vi "Parse TOML String.vi"(8 "error in (no error)":errorcluster, 11 "String":string) -> (0 "error out":errorcluster, 3 "Value":T1)   [LabVIEW 2019, in "BlueTOMLSerializer.lvlib"]
uses:
  BlueTOMLSerializer.lvlib
  Context.ctl
  State.ctl
  <vilib>/regexp/Match Regular Expression.xnode
  Value.ctl
  Key-Value Pair.ctl
  Table Context.ctl
  Array Context.ctl
  Table Array Context.ctl
  TOML Value.ctl
  Value Type.ctl
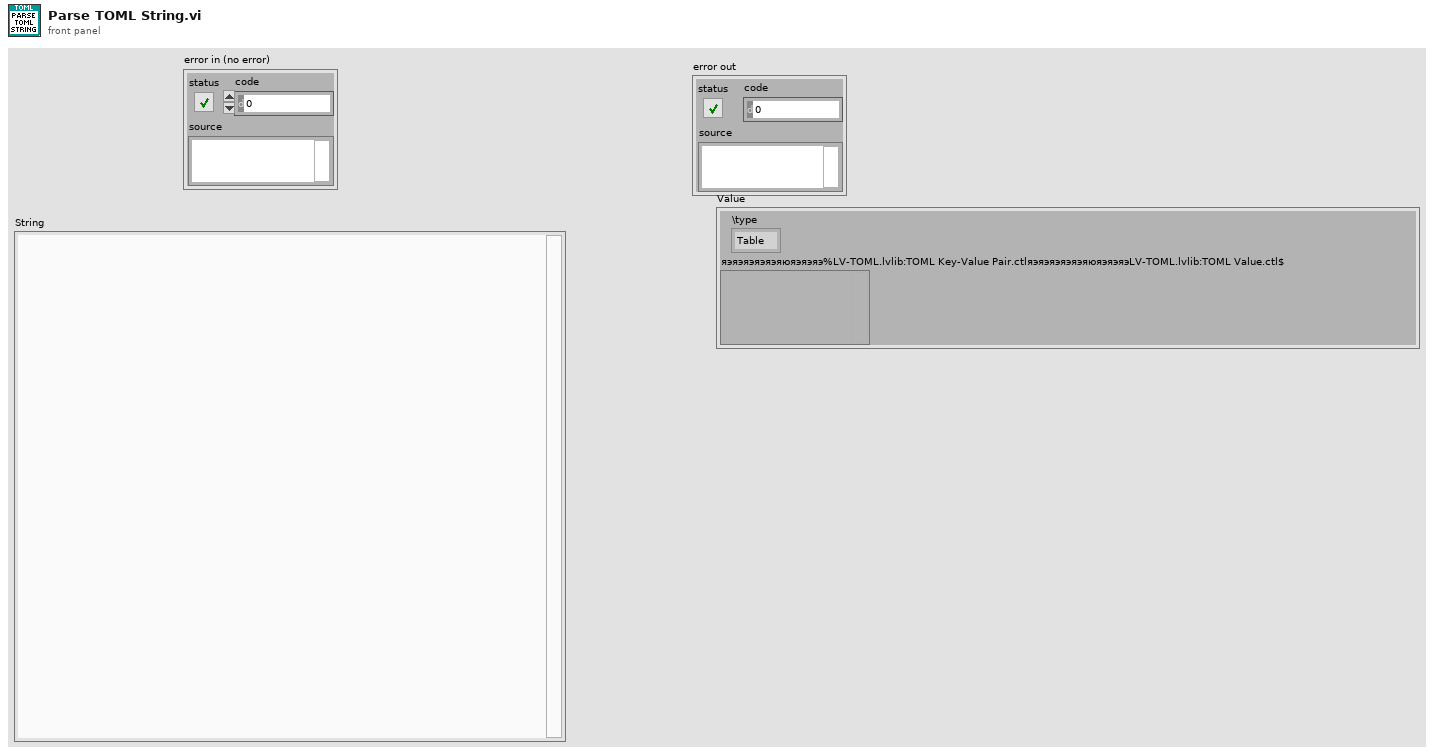
[diagram p1: front panel]
types:
  T1 = typedef "BlueTOMLSerializer.lvlib/TOML Value.ctl" = cluster{"\\type":enum16{"Table", "Array", "String", "Integer", "Float", "Boolean", "Offset Date-Time", "Local Date-Time", "Local Date", "Local Time"}, "яэяэяэяэяэяюяэяэяэ%LV-TOML.lvlib:TOML Key-Value Pair.ctlяэяэяэяэяэяюяэяэяэLV-TOML.lvlib:TOML Value.ctl$":variant}
  T2 = typedef "BlueTOMLSerializer.lvlib/Key-Value Pair.ctl" = cluster{"Key":string, "Value":T3}
  T3 = typedef "BlueTOMLSerializer.lvlib/Value.ctl" = cluster{"Type":T4, "Value":variant}
  T4 = typedef "BlueTOMLSerializer.lvlib/Value Type.ctl" = enum16{"Table", "Array", "String", "Integer", "Float", "Boolean", "Offset Date-Time", "Local Date-Time", "Local Date", "Local Time"}
  T5 = enum16{"Table", "Array", "String", "Integer", "Float", "Boolean", "Offset Date-Time", "Local Date-Time", "Local Date", "Local Time"}
  T6 = typedef "BlueTOMLSerializer.lvlib/Table Context.ctl" = cluster{"Table":T2[], "Key":string, "Defined Keys":string[]}
  T7 = typedef "BlueTOMLSerializer.lvlib/Context.ctl" = cluster{"Type":enum16{"Table", "Array", "Inline Table", "Table Array"}, "Value":variant}
  T8 = typedef "BlueTOMLSerializer.lvlib/State.ctl" = enum16{"Table", "Value", "Inline Table"}
  T9 = typedef "BlueTOMLSerializer.lvlib/Table Array Context.ctl" = cluster{"Table Array":cluster{"Table":T2[]}[], "Index":i32, "Key":string}
  T10 = typedef "BlueTOMLSerializer.lvlib/Array Context.ctl" = cluster{"Array":T3[], "Index":i32, "Empty":bool, "Type":T4}
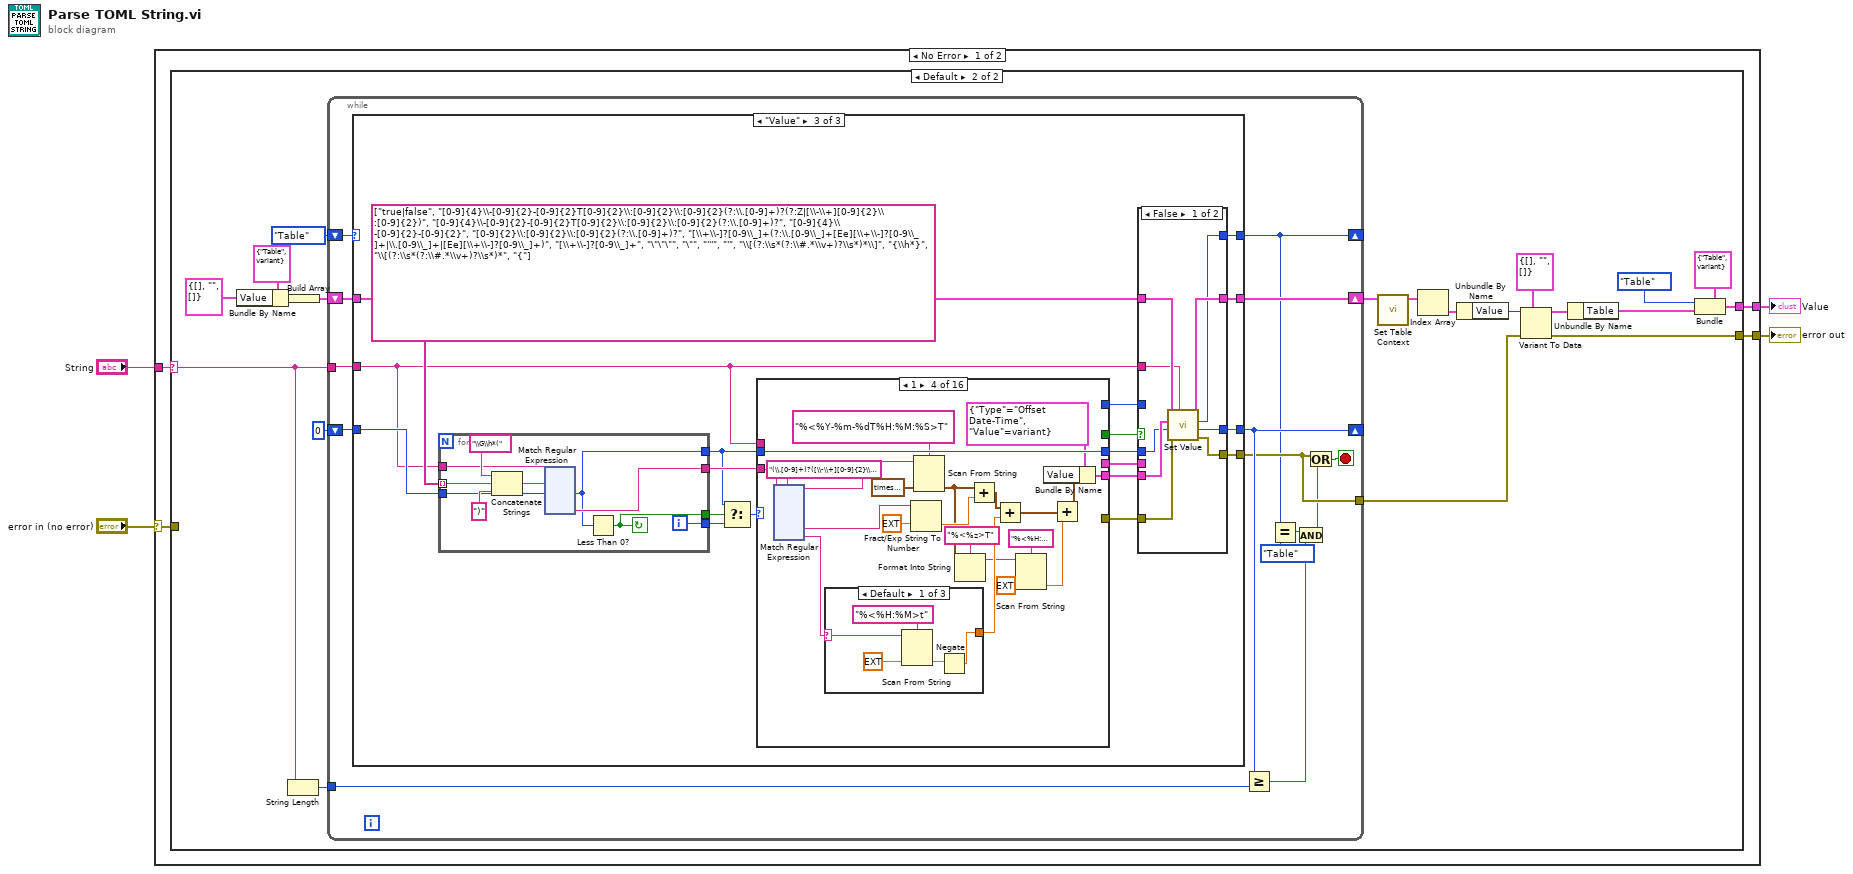
[diagram p0: block diagram]
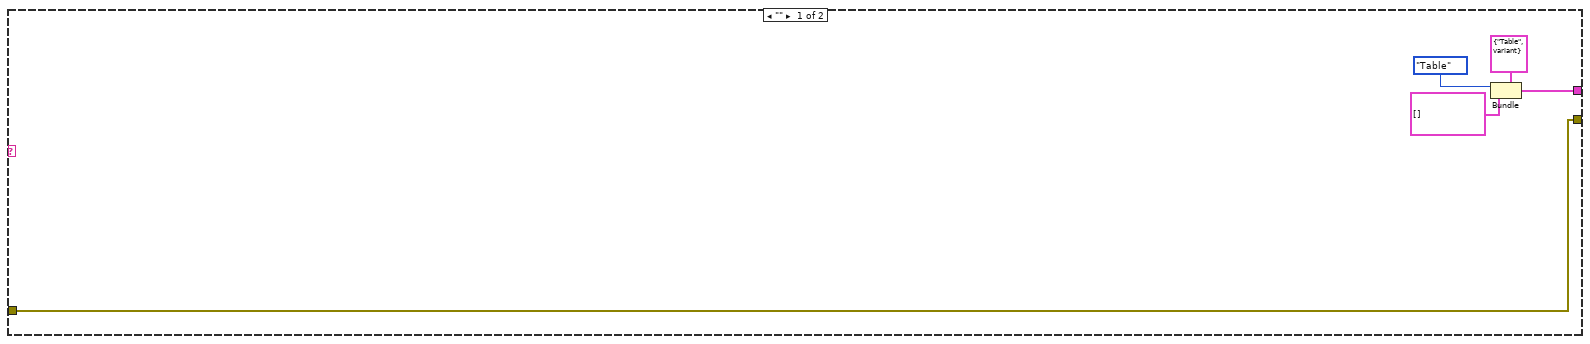
[diagram p2: hidden frame]
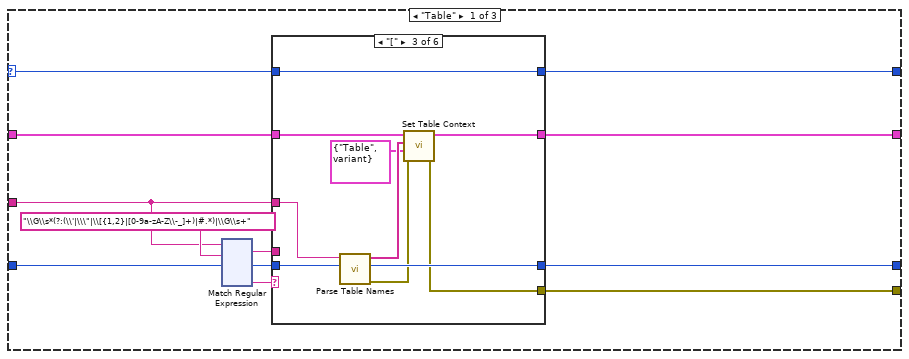
[diagram p3: hidden frame]
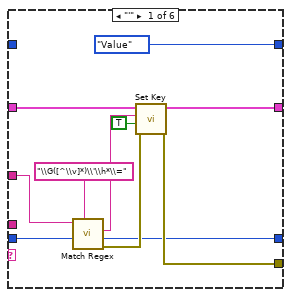
[diagram p4: hidden frame]
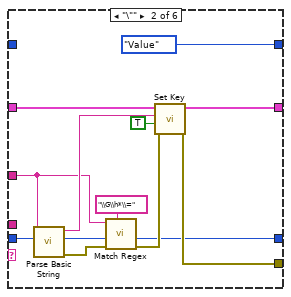
[diagram p5: hidden frame]
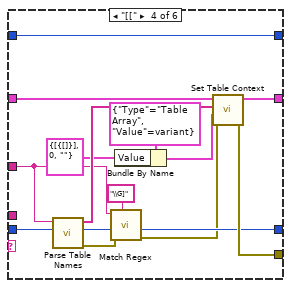
[diagram p6: hidden frame]
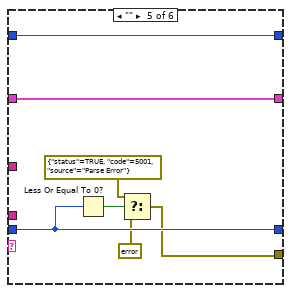
[diagram p7: hidden frame]
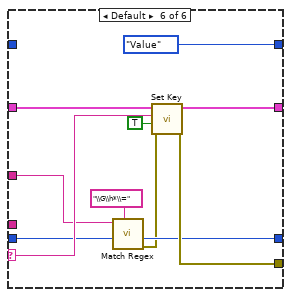
[diagram p8: hidden frame]
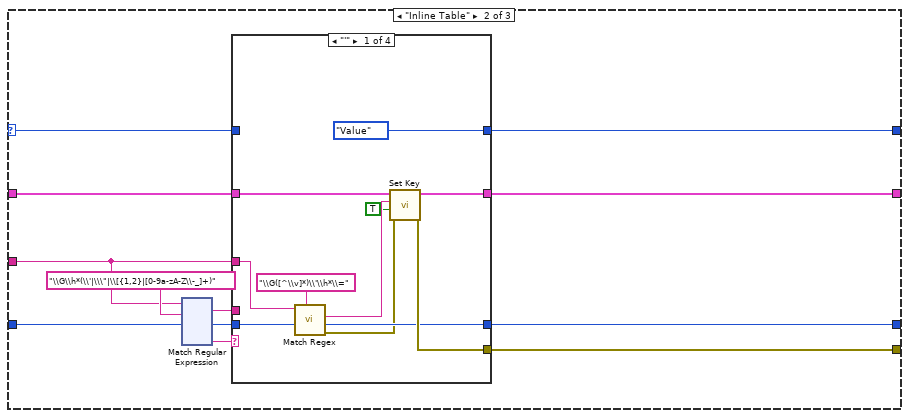
[diagram p9: hidden frame]
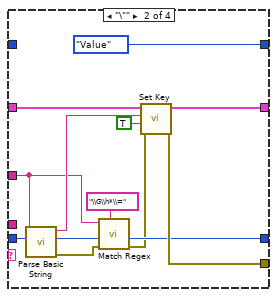
[diagram p10: hidden frame]
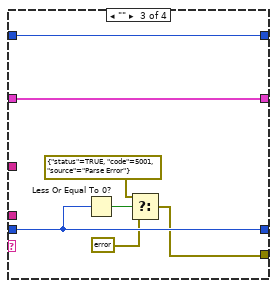
[diagram p11: hidden frame]
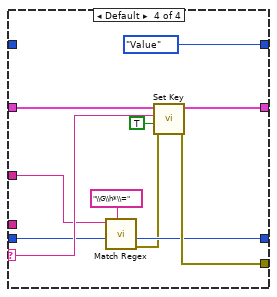
[diagram p12: hidden frame]
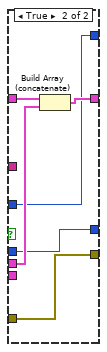
[diagram p13: hidden frame]
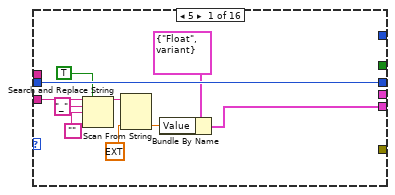
[diagram p14: hidden frame]
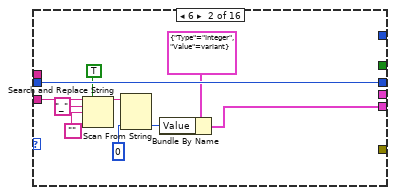
[diagram p15: hidden frame]
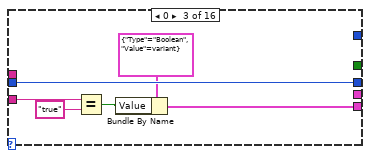
[diagram p16: hidden frame]
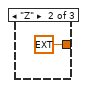
[diagram p17: hidden frame]
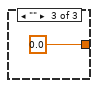
[diagram p18: hidden frame]
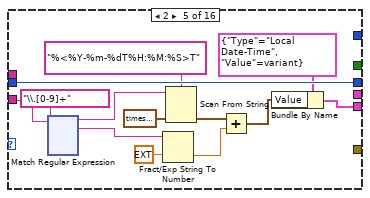
[diagram p19: hidden frame]
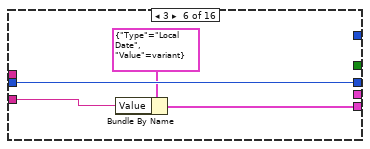
[diagram p20: hidden frame]
diagram:
  n1 = case shown="No Error" "error in (no error)" {
    selector: "error in (no error)" -> [w5 w930]
    tunnel: "String" -> [w8 _]
    tunnel: [w6 _] -> w1
    tunnel: [w7 w930] -> w3
    frame No Error {
      n2 = case shown="Default" w8 {
        selector: w8 -> [_ w31]
        tunnel: [w13 w23] -> w7
        tunnel: [w9 w18] -> w6
        tunnel: w5 -> [w13 _]
        frame "" {
          n3 = Bundle(cluster=T1 {"\\type"=enum."Table", "яэяэяэяэяэяюяэяэяэ%LV-TOML.lvlib:TOML Key-Value Pair.ctlяэяэяэяэяэяюяэяэяэLV-TOML.lvlib:TOML Value.ctl$"=variant} ("Value"), "\\type"=T5."Table" ("Type"), "яэяэяэяэяэяюяэяэяэ%LV-TOML.lvlib:TOML Key-Value Pair.ctlяэяэяэяэяэяюяэяэяэLV-TOML.lvlib:TOML Value.ctl$"=T2[] [] ("Table")) -> (w9:T1)
        }
        frame Default {
          n4 = Bundle By Name(cluster=T7 {"Type"=enum."Table", "Value"=variant} ("Context"), "Value"=T6 {"Table"=[], "Key"="", "Defined Keys"=[]} ("Table Context")) -> (w15:T7)
          n5 = String Length(string=w31) -> (length=w30:i32)
          n6 = Build Array(w15) -> (w14:T7[])
          n7 = while {
            tunnel: w31 -> [w46]
            shift-right: [w36] -> _
            shift-left: State."Table" ("State") -> [w47]
            shift-right: [w44] -> w29
            shift-left: w14 -> [w43]
            shift-right: [w39] -> _
            shift-left: 0 -> [w45]
            tunnel: w30 -> [w41]
            tunnel: [w38] -> w22
            stop <- w42 stop-if-true
            n8 = case shown="\"Value\"" w47 {
              selector: w47 -> [w55 w250 _]
              tunnel: w46 -> [w49 w244 w413]
              tunnel: w45 -> [w48 w243 w430]
              tunnel: [w56 w251 w417] -> w36
              tunnel: [w54 w249 w424] -> w44
              tunnel: w43 -> [w53 w248 w423]
              tunnel: [w57 w252 w414] -> w39
              tunnel: [w52 w247 w421] -> w38
              frame "Table" {
                n9 = xnode "Match Regular Expression"("input string"=w49, "regular expression"="\\G\\s*(?:(\\'|\\\"|\\[{1,2}|[0-9a-zA-Z\\-_]+)|#.*)|\\G\\s+", "offset (0)"=w48) -> ("whole match"=w50:string, "offset past match"=w58:i32, "submatch 1"=w51:string)  [unwired: 3 in, 3 out]
                n10 = case shown="\"[\"" w51 {
                  selector: w51 -> [_ _ _ _ _ w122]
                  tunnel: [w61 w72 w90 w99 w113 w118] -> w57
                  tunnel: w58 -> [w62 w83 w91 w107 w113 w119]
                  tunnel: [State."Value" ("State") State."Value" ("State") w93 w108 w115 State."Value" ("State")] -> w56
                  tunnel: w55 -> [_ _ w93 w108 w115 _]
                  tunnel: [w66 w79 w88 w105 w114 w123] -> w54
                  tunnel: w53 -> [w69 w80 w89 w106 w114 w124]
                  tunnel: [w67 w81 w84 w103 w109 w125] -> w52
                  tunnel: w49 -> [w63 w76 w92 w101 _ w120]
                  tunnel: w50 -> [_ _ _ _ _ _]
                  frame "'" {
                    n11 = call "Match Regex.vi"("regular expression"="\\G([^\\v]*)\\'\\h*\\=", "offset"=w62, "String"=w63) -> ("error out"=w68:errorcluster, "offset past match"=w61:i32, "submatch 1"=w64:string)  [unwired: 5 in, 1 out]
                    n12 = call "Set Key.vi"("error in (no error)"=w68, "Define"=TRUE, "Key"=w64, "Stack in"=w69) -> ("error out"=w67:errorcluster, "Stack out"=w66:T7[])  [unwired: 6 in]
                  }
                  frame "\"" {
                    n13 = call "Parse Basic String.vi"("start at"=w83, "TOML String"=w76) -> ("error out"=w74:errorcluster, "offset past match"=w75:i32, "String"=w78:string)  [unwired: 7 in]
                    n14 = call "Match Regex.vi"("regular expression"="\\G\\h*\\=", "error in (no error)"=w74, "offset"=w75, "String"=w76) -> ("error out"=w73:errorcluster, "offset past match"=w72:i32)  [unwired: 4 in, 2 out]
                    n15 = call "Set Key.vi"("error in (no error)"=w73, "Define"=TRUE, "Key"=w78, "Stack in"=w80) -> ("error out"=w81:errorcluster, "Stack out"=w79:T7[])  [unwired: 6 in]
                  }
                  frame "[" {
                    n16 = call "Parse Table Names.vi"("start at"=w91, "TOML String"=w92) -> ("error out"=w85:errorcluster, "offset past match"=w90:i32, "Table Stack"=w87:string[])  [unwired: 7 in]
                    n17 = call "Set Table Context.vi"("error in (no error)"=w85, "Context"=T7 {"Type"=enum."Table", "Value"=variant}, "Table Names"=w87, "Stack in"=w89) -> ("error out"=w84:errorcluster, "Stack out"=w88:T7[])  [unwired: 6 in]
                  }
                  frame "[[" {
                    n18 = call "Parse Table Names.vi"("start at"=w107, "TOML String"=w101) -> ("error out"=w98:errorcluster, "offset past match"=w100:i32, "Table Stack"=w104:string[])  [unwired: 7 in]
                    n19 = call "Match Regex.vi"("regular expression"="\\G]", "error in (no error)"=w98, "offset"=w100, "String"=w101) -> ("error out"=w97:errorcluster, "offset past match"=w99:i32)  [unwired: 4 in, 2 out]
                    n20 = Bundle By Name(cluster=T7 {"Type"=enum."Table Array", "Value"=variant} ("Context"), "Value"=T9 {"Table Array"=[{"Table"=[]}], "Index"=0, "Key"=""} ("Table Array Context")) -> (w95:T7)
                    n21 = call "Set Table Context.vi"("error in (no error)"=w97, "Context"=w95, "Table Names"=w104, "Stack in"=w106) -> ("error out"=w103:errorcluster, "Stack out"=w105:T7[])  [unwired: 6 in]
                  }
                  frame "" {
                    n22 = Less Or Equal To 0?(x=w113) -> (x <= 0?=w112:bool)
                    n23 = Select(t=errorcluster {"status"=TRUE, "code"=5001, "source"="Parse Error"} ("error constant"), s=w112, f=errorcluster {"status"=FALSE, "code"=0, "source"=""}) -> (s? t:f=w109:errorcluster)
                  }
                  frame Default {
                    n24 = call "Match Regex.vi"("regular expression"="\\G\\h*\\=", "offset"=w119, "String"=w120) -> ("error out"=w117:errorcluster, "offset past match"=w118:i32)  [unwired: 5 in, 2 out]
                    n25 = call "Set Key.vi"("error in (no error)"=w117, "Define"=TRUE, "Key"=w122, "Stack in"=w124) -> ("error out"=w125:errorcluster, "Stack out"=w123:T7[])  [unwired: 6 in]
                  }
                }
              }
              frame "Inline Table" {
                n26 = xnode "Match Regular Expression"("input string"=w244, "regular expression"="\\G\\h*(\\'|\\\"|\\[{1,2}|[0-9a-zA-Z\\-_]+)", "offset (0)"=w243) -> ("whole match"=w245:string, "offset past match"=w253:i32, "submatch 1"=w246:string)  [unwired: 3 in, 3 out]
                n27 = case shown="\"'\"" w246 {
                  selector: w246 -> [_ _ _ w292]
                  tunnel: [w258 w271 w284 w288] -> w252
                  tunnel: w253 -> [w259 w278 w284 w289]
                  tunnel: [State."Value" ("State") State."Value" ("State") w279 State."Value" ("State")] -> w251
                  tunnel: w250 -> [_ _ w279 _]
                  tunnel: [w262 w274 w285 w293] -> w249
                  tunnel: w248 -> [w264 w275 w285 w294]
                  tunnel: [w263 w276 w280 w295] -> w247
                  tunnel: w244 -> [w260 w270 _ w290]
                  tunnel: w245 -> [_ _ _ _]
                  frame "'" {
                    n28 = call "Match Regex.vi"("regular expression"="\\G([^\\v]*)\\'\\h*\\=", "offset"=w259, "String"=w260) -> ("error out"=w256:errorcluster, "offset past match"=w258:i32, "submatch 1"=w257:string)  [unwired: 5 in, 1 out]
                    n29 = call "Set Key.vi"("error in (no error)"=w256, "Define"=TRUE, "Key"=w257, "Stack in"=w264) -> ("error out"=w263:errorcluster, "Stack out"=w262:T7[])  [unwired: 6 in]
                  }
                  frame "\"" {
                    n30 = call "Parse Basic String.vi"("start at"=w278, "TOML String"=w270) -> ("error out"=w267:errorcluster, "offset past match"=w272:i32, "String"=w273:string)  [unwired: 7 in]
                    n31 = call "Match Regex.vi"("regular expression"="\\G\\h*\\=", "error in (no error)"=w267, "offset"=w272, "String"=w270) -> ("error out"=w268:errorcluster, "offset past match"=w271:i32)  [unwired: 4 in, 2 out]
                    n32 = call "Set Key.vi"("error in (no error)"=w268, "Define"=TRUE, "Key"=w273, "Stack in"=w275) -> ("error out"=w276:errorcluster, "Stack out"=w274:T7[])  [unwired: 6 in]
                  }
                  frame "" {
                    n33 = Less Or Equal To 0?(x=w284) -> (x <= 0?=w283:bool)
                    n34 = Select(t=errorcluster {"status"=TRUE, "code"=5001, "source"="Parse Error"} ("error constant"), s=w283, f=errorcluster {"status"=FALSE, "code"=0, "source"=""}) -> (s? t:f=w280:errorcluster)
                  }
                  frame Default {
                    n35 = call "Match Regex.vi"("regular expression"="\\G\\h*\\=", "offset"=w289, "String"=w290) -> ("error out"=w287:errorcluster, "offset past match"=w288:i32)  [unwired: 5 in, 2 out]
                    n36 = call "Set Key.vi"("error in (no error)"=w287, "Define"=TRUE, "Key"=w292, "Stack in"=w294) -> ("error out"=w295:errorcluster, "Stack out"=w293:T7[])  [unwired: 6 in]
                  }
                }
              }
              frame "Value" {
                n37 = for {
                  tunnel: string[] ["true|false", "[0-9]{4}\\-[0-9]{2}-[0-9]{2}T[0-9]{2}\\:[0-9]{2}\\:[0-9]{2}(?:\\.[0-9]+)?(?:Z|[\\-\\+][0-9]{2}\\:[0-9]{2})", "[0-9]{4}\\-[0-9]{2}-[0-9]{2}T[0-9]{2}\\:[0-9]{2}\\:[0-9]{2}(?:\\.[0-9]+)?", "[0-9]{4}\\-[0-9]{2}-[0-9]{2}", "[0-9]{2}\\:[0-9]{2}\\:[0-9]{2}(?:\\.[0-9]+)?", "[\\+\\-]?[0-9\\_]+(?:\\.[0-9\\_]+[Ee][\\+\\-]?[0-9\\_]+|\\.[0-9\\_]+|[Ee][\\+\\-]?[0-9\\_]+)", "[\\+\\-]?[0-9\\_]+", "\"\"\"", "\"", "'''", "'", "\\[(?:\\s*(?:\\#.*\\v+)?\\s*)*\\]", "{\\h*}", "\\[(?:\\s*(?:\\#.*\\v+)?\\s*)*", "{"] -> [w813] mode=indexing
                  tunnel: w413 -> [w809]
                  tunnel: w430 -> [w808]
                  tunnel: [w807] -> w426
                  tunnel: [w806] -> w425
                  tunnel: [w805] -> w429
                  tunnel: [w804] -> w428
                  i -> [w804]
                  stop <- w805 continue-if-true
                  n38 = Concatenate Strings("\\G\\h*(" ("string"), w813, ")" ("string")) -> (w810:string)
                  n39 = xnode "Match Regular Expression"("input string"=w809, "regular expression"=w810, "offset (0)"=w808) -> ("offset past match"=w806:i32, "submatch 1"=w807:string)  [unwired: 3 in, 4 out]
                  n40 = Less Than 0?(x=w806) -> (x < 0?=w805:bool)
                }
                n41 = Select(t=w425, s=w429, f=w428) -> (s? t:f=w427:i32)
                n42 = case shown="1" w427 {
                  tunnel: w426 -> [w451 w461 w471 w481 w621 w746 w750 _ _ _ _ _ _ _ _ _]
                  tunnel: w425 -> [w456 w466 w472 w494 w631 w749 w753 w755 w762 w770 w775 w779 w786 w795 w801 w803]
                  tunnel: [w456 w466 w472 w494 w631 w749 w753 w754 w761 w771 w775 w779 w783 w795 w801 w803] -> w415
                  tunnel: [_ _ _ _ _ _ _ _ _ w768 _ _ w782 _ _ errorcluster {"status"=TRUE, "code"=5001, "source"=""} ("error constant")] -> w422
                  tunnel: [w452 w462 w467 w492 w629 w747 w751 w758 w764 w772 w776 w780 w788 _ _ _] -> w420
                  tunnel: w413 -> [_ _ _ _ _ _ _ w757 w763 w767 _ _ w785 _ _ _]
                  tunnel: [_ _ _ _ _ _ _ _ _ _ _ _ _ TRUE TRUE _] -> w419
                  tunnel: [_ _ _ _ _ _ _ _ _ _ _ _ _ w791 w798 _] -> w418
                  tunnel: [_ _ _ _ _ _ _ _ _ _ _ _ _ State."Value" ("State") State."Inline Table" ("State") _] -> w416
                  frame 5 {
                    n43 = Search and Replace String(replace all?=TRUE ("replace all? (F)"), input string=w451, search string="_", replace string="") -> (result string=w450:string)  [unwired: 4 in, 3 out]
                    n44 = Scan From String(input string=w450, default 1=ext 0.0 ("default value 1")) -> (output 1=w454:ext)  [unwired: 3 in, 3 out]
                    n45 = Bundle By Name(cluster=T3 {"Type"=enum."Float", "Value"=variant} ("Value"), "Value"=w454) -> (w452:T3)
                  }
                  frame 6 {
                    n46 = Search and Replace String(replace all?=TRUE ("replace all? (F)"), input string=w461, search string="_", replace string="") -> (result string=w460:string)  [unwired: 4 in, 3 out]
                    n47 = Scan From String(input string=w460, default 1=i64 0 ("default value 1")) -> (output 1=w464:i64)  [unwired: 3 in, 3 out]
                    n48 = Bundle By Name(cluster=T3 {"Type"=enum."Integer", "Value"=variant} ("Value"), "Value"=w464) -> (w462:T3)
                  }
                  frame 0 {
                    n49 = Equal?(x=w471, y="true") -> (x = y?=w468:bool)
                    n50 = Bundle By Name(cluster=T3 {"Type"=enum."Boolean", "Value"=variant} ("Value"), "Value"=w468) -> (w467:T3)
                  }
                  frame 1 {
                    n51 = xnode "Match Regular Expression"("input string"=w481, "regular expression"="(\\.[0-9]+)?([\\-\\+][0-9]{2}\\:[0-9]{2}|Z)$") -> ("before match"=w486:string, "submatch 1"=w485:string, "submatch 2"=w483:string)  [unwired: 4 in, 4 out]
                    n52 = case shown="Default" w483 {
                      selector: w483 -> [w499 _ _]
                      tunnel: [w495 ext 0.0 0.0] -> w482
                      frame Default {
                        n53 = Scan From String(format string="%<%H:%M>t", input string=w499, default 1=ext 0.0 ("default value 1")) -> (output 1=w496:ext)  [unwired: 2 in, 3 out]
                        n54 = Negate(x=w496) -> (-x=w495:ext)
                      }
                      frame "Z" {
                      }
                      frame "" {
                      }
                    }
                    n55 = Fract/Exp String To Number(string=w485, default (0 dbl)=ext 0.0 ("default (0 DBL)")) -> (number=w487:ext)  [unwired: 2 in, 1 out]
                    n56 = Scan From String(format string="%<%Y-%m-%dT%H:%M:%S>T", input string=w486, default 1=timestamp(0 s since 1904-01-01)) -> (output 1=w473:timestamp)  [unwired: 2 in, 3 out]
                    n57 = Format Into String(format string="%<%z>T", w473) -> (resulting string=w476:string)  [unwired: 2 in, 1 out]
                    n58 = Add(x=w473, y=w487) -> (x+y=w484:timestamp)
                    n59 = Add(x=w484, y=w482) -> (x+y=w480:timestamp)
                    n60 = Scan From String(format string="%<%H:%M:%S>t", input string=w476, default 1=ext 0.0 ("default value 1")) -> (output 1=w475:ext)  [unwired: 2 in, 3 out]
                    n61 = Add(x=w480, y=w475) -> (x+y=w474:timestamp)
                    n62 = Bundle By Name(cluster=T3 {"Type"=enum."Offset Date-Time", "Value"=variant} ("Value"), "Value"=w474) -> (w492:T3)
                  }
                  frame 2 {
                    n63 = xnode "Match Regular Expression"("input string"=w621, "regular expression"="\\.[0-9]+") -> ("before match"=w622:string, "whole match"=w619:string)  [unwired: 4 in, 3 out]
                    n64 = Fract/Exp String To Number(string=w619, default (0 dbl)=ext 0.0 ("default (0 DBL)")) -> (number=w623:ext)  [unwired: 2 in, 1 out]
                    n65 = Scan From String(format string="%<%Y-%m-%dT%H:%M:%S>T", input string=w622, default 1=timestamp(0 s since 1904-01-01)) -> (output 1=w624:timestamp)  [unwired: 2 in, 3 out]
                    n66 = Add(x=w624, y=w623) -> (x+y=w620:timestamp)
                    n67 = Bundle By Name(cluster=T3 {"Type"=enum."Local Date-Time", "Value"=variant} ("Value"), "Value"=w620) -> (w629:T3)
                  }
                  frame 3 {
                    n68 = Bundle By Name(cluster=T3 {"Type"=enum."Local Date", "Value"=variant} ("Value"), "Value"=w746) -> (w747:T3)
                  }
                  frame 4 {
                    n69 = Bundle By Name(cluster=T3 {"Type"=enum."Local Time", "Value"=variant} ("Value"), "Value"=w750) -> (w751:T3)
                  }
                  frame 7 {
                    n70 = call "Parse Multiline Basic String.vi"("start at"=w755, "TOML String"=w757) -> ("offset past match"=w754:i32, "String"=w756:string)  [unwired: 7 in, 1 out]
                    n71 = Bundle By Name(cluster=T3 {"Type"=enum."String", "Value"=variant} ("Value"), "Value"=w756) -> (w758:T3)
                  }
                  frame 8 {
                    n72 = call "Parse Basic String.vi"("start at"=w762, "TOML String"=w763) -> ("offset past match"=w761:i32, "String"=w760:string)  [unwired: 7 in, 1 out]
                    n73 = Bundle By Name(cluster=T3 {"Type"=enum."String", "Value"=variant} ("Value"), "Value"=w760) -> (w764:T3)
                  }
                  frame 10 {
                    n74 = call "Match Regex.vi"("regular expression"="\\G([^\\v]*)\\'", "offset"=w770, "String"=w767) -> ("error out"=w768:errorcluster, "offset past match"=w771:i32, "submatch 1"=w769:string)  [unwired: 5 in, 1 out]
                    n75 = Bundle By Name(cluster=T3 {"Type"=enum."String", "Value"=variant} ("Value"), "Value"=w769) -> (w772:T3)
                  }
                  frame 11 {
                    n76 = Bundle By Name(cluster=T3 {"Type"=enum."Array", "Value"=variant} ("Value"), "Value"=T3[] []) -> (w776:T3)
                  }
                  frame 12 {
                    n77 = Bundle By Name(cluster=T3 {"Type"=enum."Table", "Value"=variant} ("Value"), "Value"=T2[] []) -> (w780:T3)
                  }
                  frame 9 {
                    n78 = call "Match Regex.vi"("regular expression"="\\G(?:\\r\\h*|\\n\\h*|\\r\\n\\h*)?((?s:.)*?)'''", "offset"=w786, "String"=w785) -> ("error out"=w782:errorcluster, "offset past match"=w783:i32, "submatch 1"=w787:string)  [unwired: 5 in, 1 out]
                    n79 = Bundle By Name(cluster=T3 {"Type"=enum."String", "Value"=variant} ("Value"), "Value"=w787) -> (w788:T3)
                  }
                  frame 13 {
                    n80 = Bundle By Name(cluster=T7 {"Type"=enum."Array", "Value"=variant} ("Context"), "Value"=T10 {"Array"=[], "Index"=0, "Empty"=TRUE, "Type"=enum."Table"} ("Array Context")) -> (w791:T7)
                  }
                  frame 14 {
                    n81 = Bundle By Name(cluster=T7 {"Type"=enum."Inline Table", "Value"=variant} ("Context"), "Value"=T6 {"Table"=[], "Key"="", "Defined Keys"=[]} ("Table Context")) -> (w798:T7)
                  }
                  frame Default {
                  }
                }
                n82 = case shown="False" w419 {
                  tunnel: [w440 w444] -> w424
                  tunnel: w423 -> [w439 w445]
                  tunnel: w422 -> [w438 w446]
                  tunnel: [w437 w446] -> w421
                  tunnel: w420 -> [w436 _]
                  tunnel: w418 -> [_ w443]
                  tunnel: [w435 w442] -> w417
                  tunnel: w416 -> [_ w442]
                  tunnel: w415 -> [w434 w441]
                  tunnel: [w433 w441] -> w414
                  tunnel: w413 -> [w432 _]
                  frame False {
                    n83 = call "Set Value.vi"("TOML string"=w432, "error in (no error)"=w438, "start position"=w434, "Value"=w436, "Context in"=w439) -> ("error out"=w437:errorcluster, "offset past match"=w433:i32, "State"=w435:T8, "Context out"=w440:T7[])  [unwired: 3 in]
                  }
                  frame True {
                    n84 = Build Array (concatenate)(w445, w443) -> (w444:T7[])
                  }
                }
              }
            }
            n85 = Greater Or Equal?(x=w39, y=w41) -> (x >= y?=w40:bool)
            n86 = Equal?(x=w36, y=State."Table") -> (x = y?=w34:bool)
            n87 = And(x=w34, y=w40) -> (x .and. y?=w37:bool)
            n88 = Or(x=w38, y=w37) -> (x .or. y?=w42:bool)
          }
          n89 = call "Set Table Context.vi"("Stack in"=w29) -> ("Stack out"=w28:T7[])  [unwired: 9 in, 1 out]
          n90 = Index Array(array=w28) -> (element=w26:T7)  [unwired: 1 in]
          n91 = Unbundle By Name(w26) -> ("Value"=w25:variant)
          n92 = Variant To Data(error in=w22, type=T6 {"Table"=[], "Key"="", "Defined Keys"=[]} ("Table Context"), Variant=w25) -> (data=w24:T6, error out=w23:errorcluster)
          n93 = Unbundle By Name(w24) -> ("Table"=w19:T2[])
          n94 = Bundle(cluster=T1 {"\\type"=enum."Table", "яэяэяэяэяэяюяэяэяэ%LV-TOML.lvlib:TOML Key-Value Pair.ctlяэяэяэяэяэяюяэяэяэLV-TOML.lvlib:TOML Value.ctl$"=variant} ("Value"), "\\type"=T5."Table" ("Type"), "яэяэяэяэяэяюяэяэяэ%LV-TOML.lvlib:TOML Key-Value Pair.ctlяэяэяэяэяэяюяэяэяэLV-TOML.lvlib:TOML Value.ctl$"=w19) -> (w18:T1)
        }
      }
    }
    frame Error {
    }
  }
  "error out" <- w3
  "Value" <- w1
